vi "sweep_Gadi.vi"(0 "Stop  Frequency (1000.0 Hz)":dbl=1000.0 format="%#.6g", 1 "Start Frequency (100.0 Hz)":dbl=100.0 format="%#.6g", 2 "VISA resource name in":refnum<visa-resource-name>="K-33511B-03409", 3 "error in (no error)":errorcluster, 4 "Sweep Time (1.00 s)":dbl=1.0 format="%#.6g") -> ()   [LabVIEW 2018]
uses:
  <instrlib>/Agilent 33XXX Series/Agilent 33XXX Series.lvlib
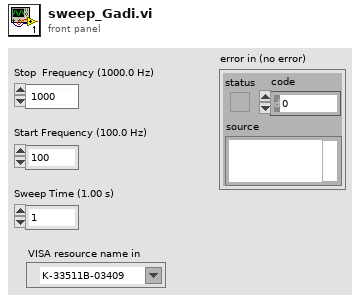
[diagram p1: front panel]
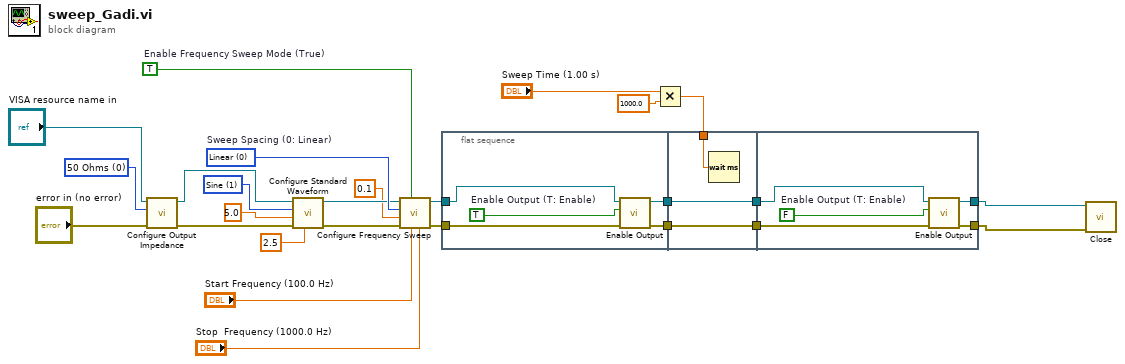
[diagram p0: block diagram]
diagram:
  w5 = u16 0 items=["50 Ohms", "High Impedance", "User Defined"] ("Impedance (0: 50 Ohms)")
  w15 = u16 1 items=["DC", "Sine", "Square", "Triangle", "Ramp", "Pulse", "Noise", "Sinc", "Negative Ramp", "Exponential Rise", "Exponential Fall", "Cardiac"] ("Waveform Function (1: Sine)")
  w18 = u16 0 items=["Linear", "Logarithmic"]  # Sweep Spacing (0: Linear)
  w12 = TRUE  # Enable Frequency Sweep Mode (True)
  n1 = call <instrlib>:"Configure Output Impedance.vi"("error in (no error)"="error in (no error)", "Impedance (0: 50 Ohms)"=w5, "VISA resource name"="VISA resource name in") -> ("error out"=w6:errorcluster, "VISA resource name out"=w7:refnum<visa-resource-name>)  [unwired: 7 in]
  n2 = call <instrlib>:"Configure Standard Waveform.vi"("DC Offset (0.00 V)"=2.5, "error in (no error)"=w6, "Amplitude (1)"=5.0 ("Amplitude (1 Vpp)"), "Waveform Function (1: Sine)"=w15, "VISA resource name"=w7) -> ("error out"=w9:errorcluster, "VISA resource name out"=w10:refnum<visa-resource-name>)  [unwired: 5 in]
  n3 = call <instrlib>:"Configure Frequency Sweep.vi"("Stop  Frequency (1000.0 Hz)"="Stop  Frequency (1000.0 Hz)", "Start Frequency (100.0 Hz)"="Start Frequency (100.0 Hz)", "Enable Frequency Sweep Mode (T: Enable)"=w12, "error in (no error)"=w9, "Sweep Time (1.00 s)"=0.1, "Sweep Spacing (0: Linear)"=w18, "VISA resource name"=w10) -> ("error out"=w17:errorcluster, "VISA resource name out"=w16:refnum<visa-resource-name>)  [unwired: 3 in]
  n4 = flat-sequence {
    tunnel: w16 -> [w31]
    tunnel: w17 -> [w30]
    tunnel: [w28] -> w26
    tunnel: [w27] -> w25
    tunnel: w22 -> [w34]
    tunnel: [w33] -> w24
    tunnel: w26 -> [w33]
    tunnel: [w32] -> w23
    tunnel: w25 -> [w32]
    tunnel: w24 -> [w38]
    tunnel: w23 -> [w37]
    tunnel: [w36] -> w1
    tunnel: [w35] -> w2
    frame #0 {
      w29 = TRUE  # Enable Output (T: Enable)
      n5 = call <instrlib>:"Enable Output.vi"("error in (no error)"=w30, "Enable Output  (T: Enable)"=w29, "VISA resource name"=w31) -> ("error out"=w27:errorcluster, "VISA resource name out"=w28:refnum<visa-resource-name>)  [unwired: 7 in]
    }
    frame #1 {
      n6 = Wait (ms)(milliseconds to wait=w34) -> ()  [unwired: 1 out]
    }
    frame #2 {
      w39 = FALSE  # Enable Output (T: Enable)
      n7 = call <instrlib>:"Enable Output.vi"("error in (no error)"=w37, "Enable Output  (T: Enable)"=w39, "VISA resource name"=w38) -> ("error out"=w35:errorcluster, "VISA resource name out"=w36:refnum<visa-resource-name>)  [unwired: 7 in]
    }
  }
  n8 = Multiply(x="Sweep Time (1.00 s)", y=1000.0) -> (x*y=w22:dbl)
  n9 = call <instrlib>:"Close.vi"("error in (no error)"=w2, "VISA resource name"=w1) -> ()  [unwired: 9 in, 1 out]
